vi "_array_shuffle.vi"(10 "total number":dbl, 11 "input array":dbl[](array[numeric])) -> (3 "output array":dbl[](array[numeric]))   [LabVIEW 2024]
uses:
  <vilib>/Analysis/1siggen.llb/Riffle Array (DBL) (obs 2012).vi
  <vilib>/Analysis/NI_AALBase.lvlib
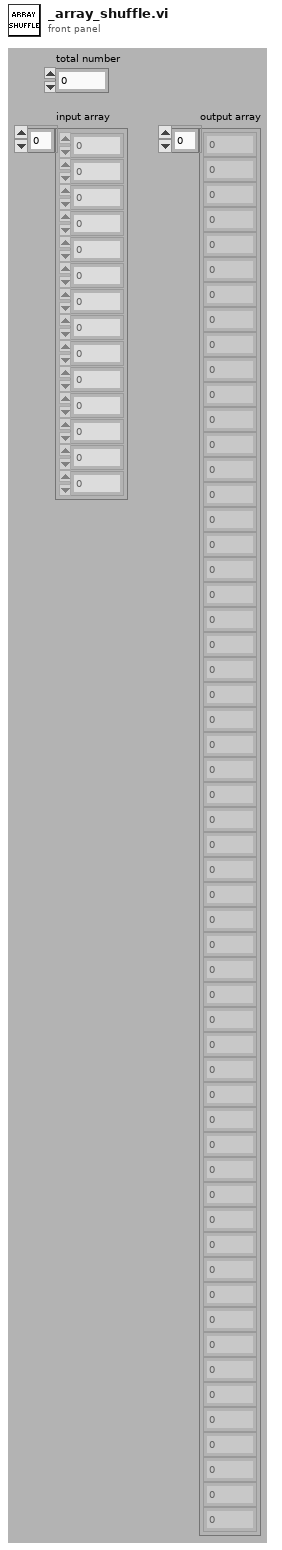
[diagram p1: front panel]
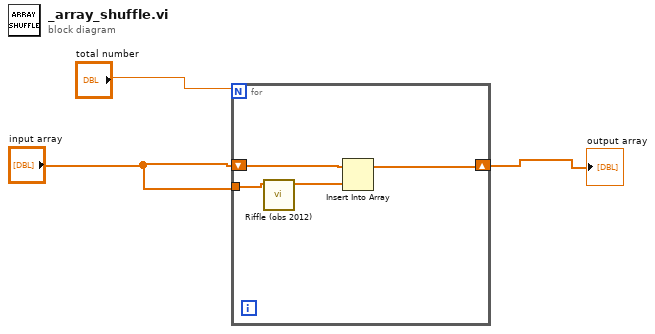
[diagram p0: block diagram]
diagram:
  n1 = for {
    N: "total number" -> [_]
    shift-right: [w7] -> w3
    shift-left: "input array" -> [w6]
    tunnel: "input array" -> [w5]
    n2 = call-poly <vilib>:"Riffle (obs 2012).vi"("X"=w5) -> ("Riffled {X}"=w4:dbl[])  [unwired: 8 in, 2 out]
    n3 = Insert Into Array(array=w6, new element=w4) -> (w7:dbl[])  [unwired: 1 in]
  }
  "output array" <- w3
